vi "set_process_layer_parameters_subset.vi"(6 "Layer number":u8, 8 "error in (no error)":errorcluster, 9 "Process number":u8, 10 "Controls[]":refnum<vi>[](array[refnum]), 11 "VISA resource name":refnum<visa-resource-name>) -> (0 "error out":errorcluster, 3 "VISA Refnum out":refnum<visa-resource-name>)   [LabVIEW 2018]
uses:
  Low Level/process_layer_parameter_ring.ctl
panel:
  in  "Process layer parameter":T1 items=["Material", "Final Thick (kA)", "Thick Limit (kA)", "Crucible", "CoDep", "Ratio Cntrl (%)"]
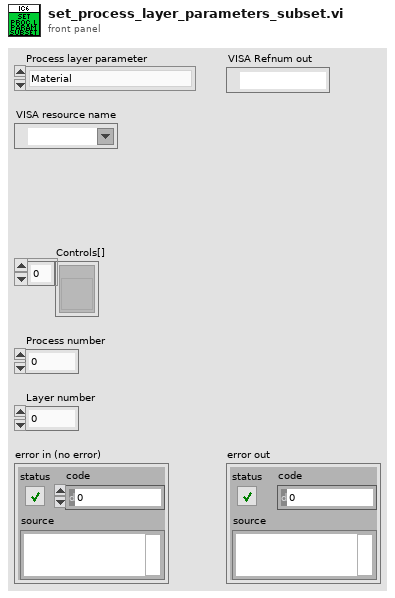
[diagram p1: front panel]
types:
  T1 = typedef "process_layer_parameter_ring.ctl" = u16
  T2 = typedef "LVStringsAndValuesArrayTypeDef_U16.ctl" = cluster{"String":string, "Value":u16}[]
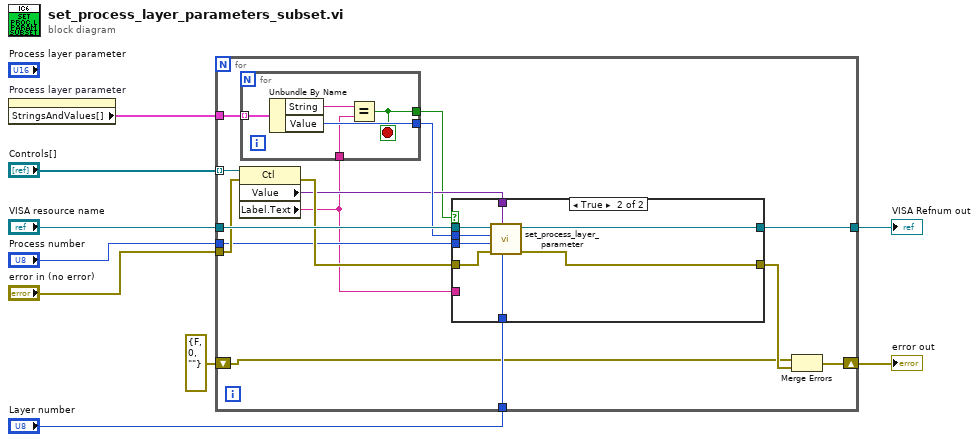
[diagram p0: block diagram]
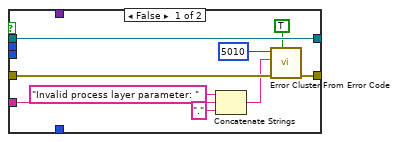
[diagram p2: hidden frame]
diagram:
  n1 = property on="Process layer parameter" class="Ring (strict)"() -> ("StringsAndValues[]"=w7:T2)  [unwired: 2 in, 2 out]
  n2 = for {
    tunnel: "VISA resource name" -> [w24]
    tunnel: [w23] -> w4
    tunnel: "error in (no error)" -> [w21]
    tunnel: "Process number" -> [w15]
    tunnel: w7 -> [w19]
    tunnel: "Controls[]" -> [w22] mode=indexing
    tunnel: "Layer number" -> [w17]
    shift-right: [w12] -> w1
    shift-left: errorcluster {"status"=FALSE, "code"=0, "source"=""} ("error IO") -> [w11]
    n3 = property class="Ctl"(reference=w22, error in=w21) -> (error out=w20:errorcluster, "Value"=w16:variant, "Label.Text"=w10:string)  [unwired: 1 out]
    n4 = for {
      tunnel: w19 -> [w46] mode=indexing
      tunnel: [w45] -> w18
      tunnel: w10 -> [w43]
      tunnel: [w42] -> w14
      stop <- w42 stop-if-true
      n5 = Unbundle By Name(w46) -> ("String"=w44:string, "Value"=w45:u16)
      n6 = Equal?(x=w44, y=w43) -> (x = y?=w42:bool)
    }
    n7 = case shown="True" w14 {
      tunnel: w24 -> [w33 w41]
      tunnel: [w33 w40] -> w23
      tunnel: w20 -> [w32 w39]
      tunnel: w18 -> [_ w38]
      tunnel: w17 -> [_ w37]
      tunnel: w16 -> [_ w36]
      tunnel: w15 -> [_ w35]
      tunnel: [w31 w34] -> w13
      tunnel: w10 -> [w26 _]
      frame False {
        n8 = Concatenate Strings("Invalid process layer parameter: " ("error message (\"\")"), w26, "." ("string")) -> (w25:string)
        n9 = call <vilib>:"Error Cluster From Error Code.vi"("show call chain? (False)"=TRUE, "error in (no error)"=w32, "error message (\"\")"=w25, "error code (0)"=5010) -> ("error out"=w31:errorcluster)  [unwired: 5 in]
      }
      frame True {
        n10 = call "set_process_layer_parameter.vi"("Layer number"=w37, "Parameter value"=w36, "error in (no error)"=w39, "Process number"=w35, "Process layer parameter"=w38, "VISA resource name"=w41) -> ("error out"=w34:errorcluster, "VISA resource name out"=w40:refnum<visa-resource-name>)  [unwired: 4 in]
      }
    }
    n11 = Merge Errors(w11, w13) -> (w12:errorcluster)
  }
  "error out" <- w1
  "VISA Refnum out" <- w4
